vi "test_PhotonCamera_EmptyResult.vi"(8 "error in (no error)":errorcluster) -> (0 "error out":errorcluster, 3 "Test Passed":bool)   [LabVIEW 2019]
uses:
  <vilib>/Rock Robotics/WPI/ThirdParty/PhotonVisionLib/PhotonVisionLib.lvlib
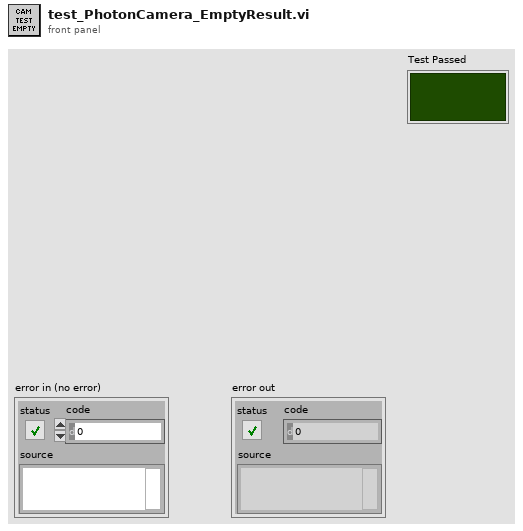
[diagram p1: front panel]
types:
  T1 = typedef "PhotonVisionLib.lvlib/PhotonPipelineResult_REF.ctl" = refnum<data-value>
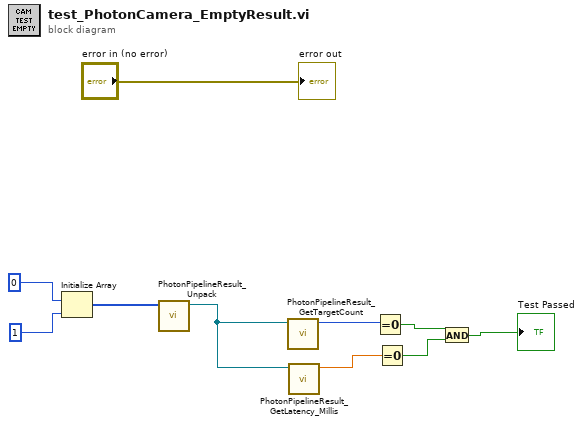
[diagram p0: block diagram]
diagram:
  n1 = Initialize Array(u8 0 ("Byte"), 1 ("dimension size")) -> (w7:u8[])
  n2 = call <vilib>:"PhotonPipelineResult_Unpack.vi"("RawData"=w7) -> ("PhotonPipelineResult_REF"=w3:T1)  [unwired: 10 in]
  n3 = call <vilib>:"PhotonPipelineResult_GetTargetCount.vi"("PhotonPipelineResult_REF"=w3) -> ("TargetCount"=w2:i32)  [unwired: 10 in]
  n4 = call <vilib>:"PhotonPipelineResult_GetLatency_Millis.vi"("PhotonPipelineResult_REF"=w3) -> ("Latency_MilliSec"=w1:dbl)  [unwired: 9 in, 1 out]
  n5 = Equal To 0?(x=w2) -> (x = 0?=w6:bool)
  n6 = Equal To 0?(x=w1) -> (x = 0?=w5:bool)
  n7 = And(x=w6, y=w5) -> (x .and. y?=→"Test Passed":bool)
  "error out" <- "error in (no error)"
